vi "单轴运动.vi"() -> ()   [LabVIEW 2011]
uses:
  <userlib>/LTDMC/LTDMC.lvlib
panel:
  in  "停止速度":dbl=100.0
  out "运行曲线图 2":cluster{dbl[], i32[]}[](graph)
  out "运行时间":dbl
  out "当前状态":string
  out "当前速度":dbl
  out "当前位置":i32
  out "运行曲线图":cluster{dbl[], dbl[]}[](graph)
  in  "在线变位":bool
  in  "变位的位置值":i32=21000
  in  "S段时间s":dbl
  in  "减速时间s":dbl=0.5
  in  "加速时间s":dbl=0.5
  in  "运行速度":dbl=100000.0
  in  "起始速度":dbl=500.0
  in  "变速的速度值":dbl=1500.0
  in  "运动模式":enum32{"相对", "绝对"}(radio)
  in  "运动距离":i32=300000
  in  "运动方式":enum32{"点位", "连续"}(radio)
  in  "运动方向":enum32{"正向", "反向"}(radio)
  in  "在线变速":bool
  in  "退出":bool
  in  "紧急停止":bool
  in  "减速停止":bool
  in  "运行":bool
  in  "轴号选择":enum32{"X轴", "Y轴", "Z轴", "C轴"}(radio)
  in  "脉冲清零":bool
  in  "卡号选择":u16(ring) items=["0", "1"]
  out "init":bool
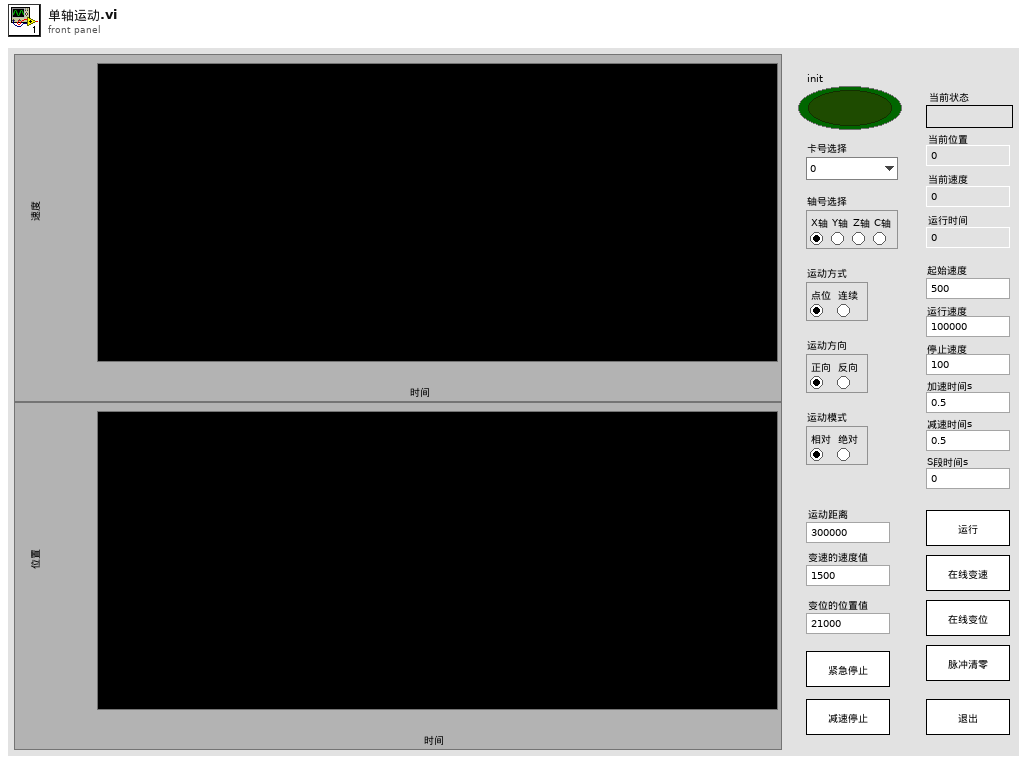
[diagram p1: front panel]
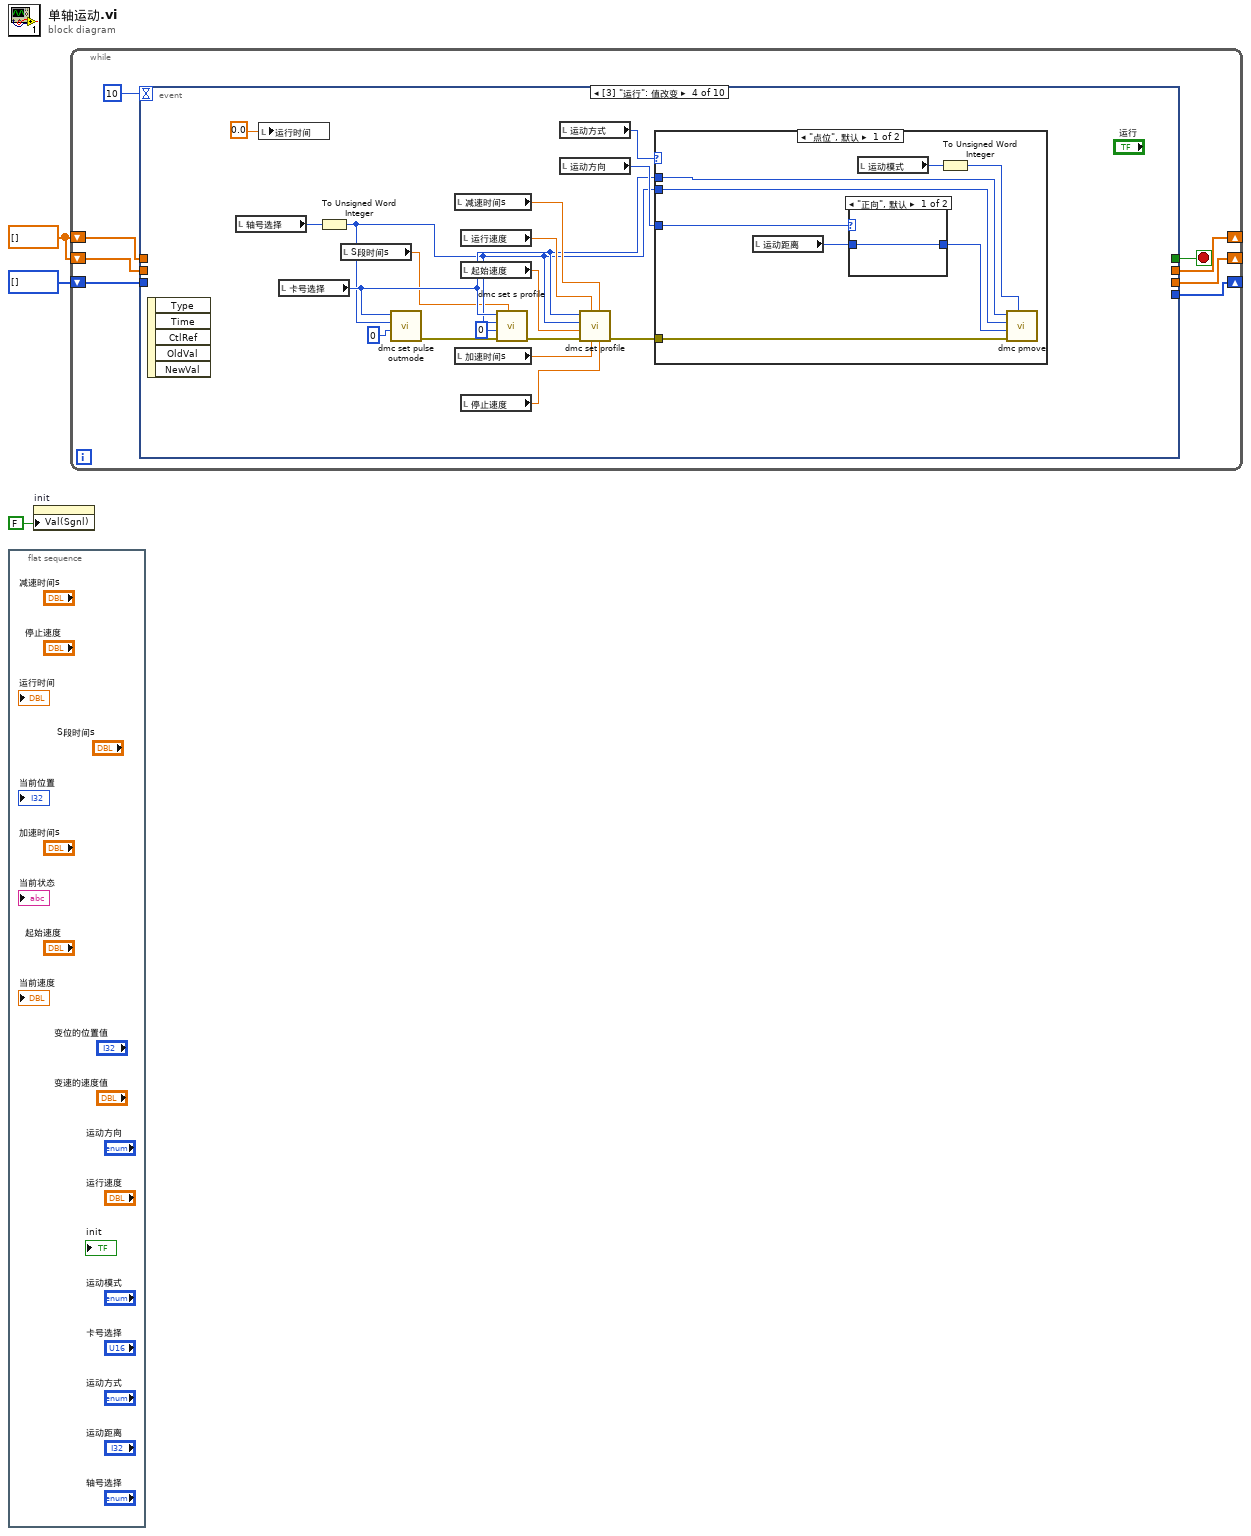
[diagram p0: block diagram]
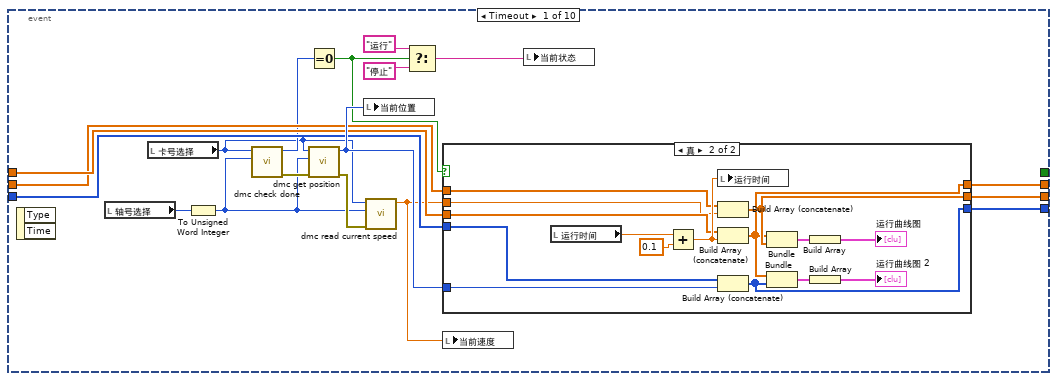
[diagram p2: hidden frame]
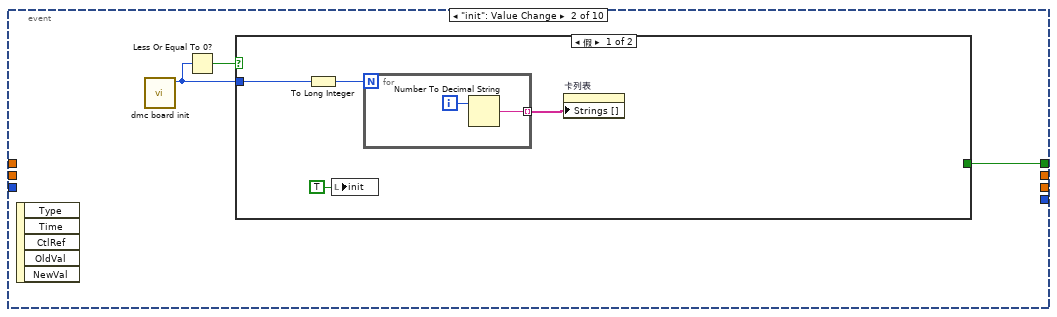
[diagram p4: hidden frame]
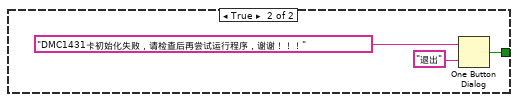
[diagram p5: hidden frame]
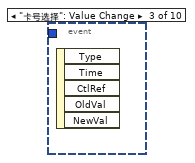
[diagram p6: hidden frame]
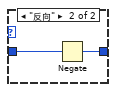
[diagram p7: hidden frame]
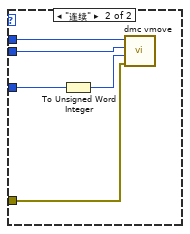
[diagram p8: hidden frame]
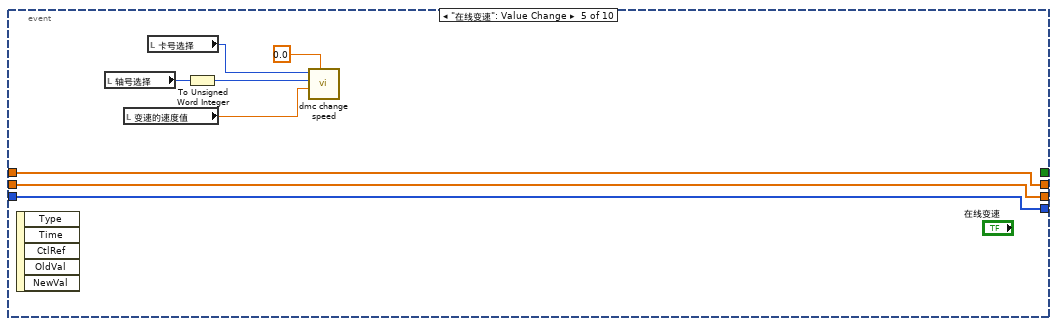
[diagram p9: hidden frame]
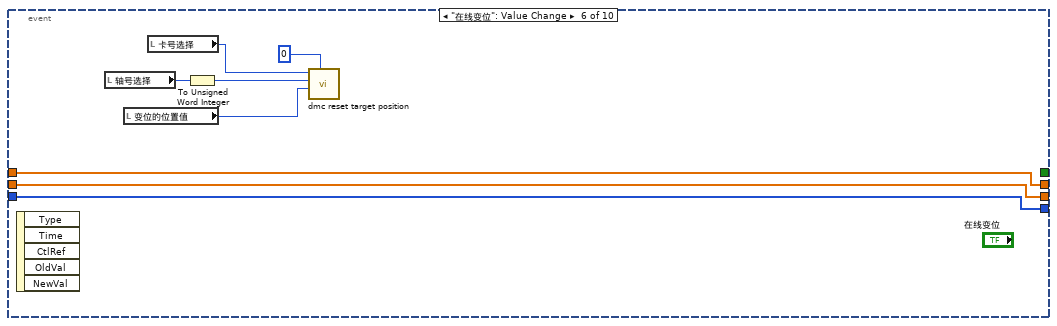
[diagram p10: hidden frame]
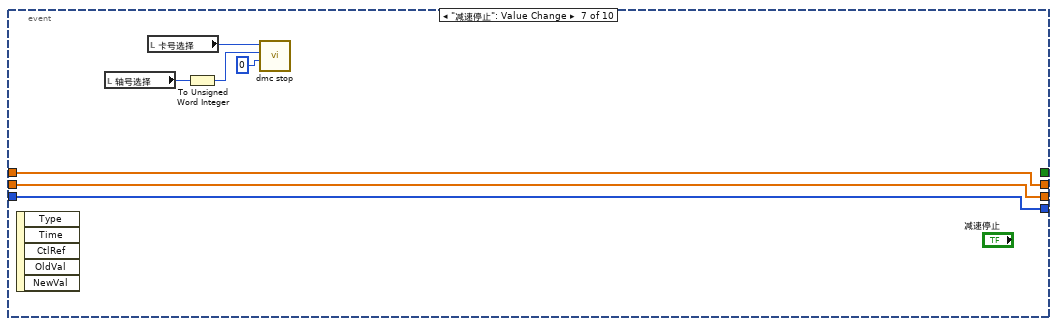
[diagram p11: hidden frame]
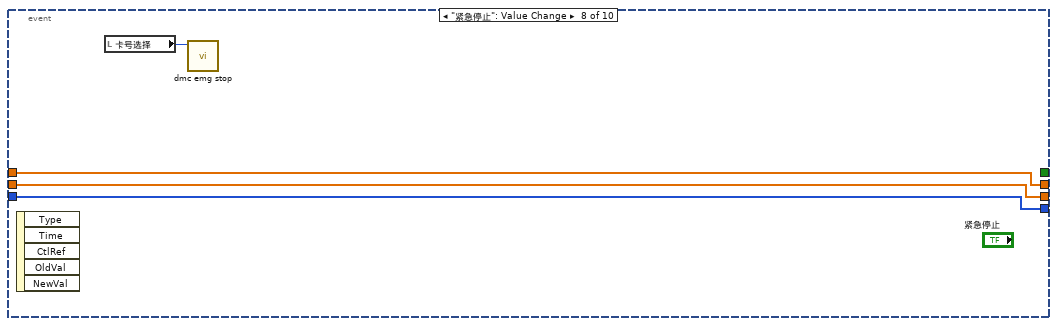
[diagram p12: hidden frame]
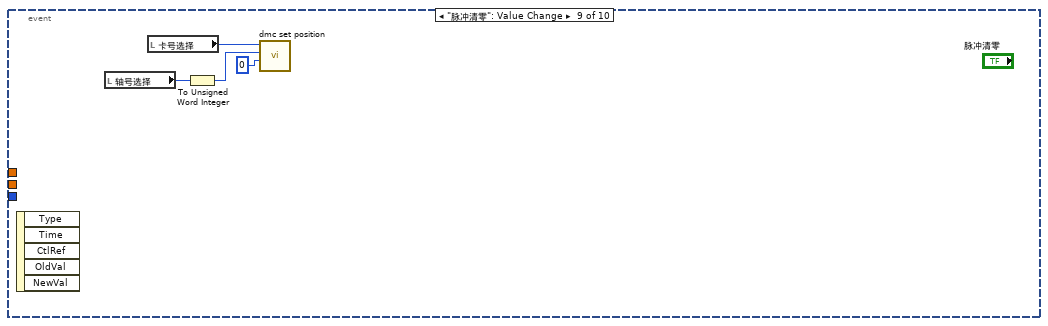
[diagram p13: hidden frame]
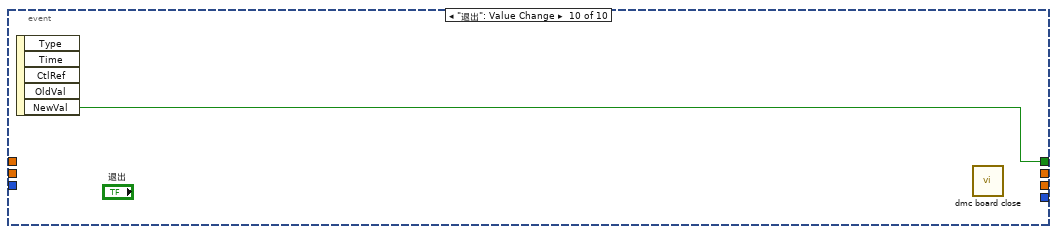
[diagram p14: hidden frame]
diagram:
  w1 = dbl[] []
  n1 = flat-sequence {
    frame #0 {
    }
  }
  n2 = property on="init" class="Bool (严格)"("Val(Sgnl)"=FALSE ("值(信号)")) -> ()  [unwired: 2 in, 2 out]
  n3 = while {
    shift-right: [w9] -> _
    shift-left: w1 -> [w8]
    shift-right: [w7] -> _
    shift-left: i32[] [] -> [w6]
    shift-right: [w4] -> _
    shift-left: w1 -> [w5]
    stop <- w11 stop-if-true
    n4 = event shown="[3] \"运行\": 值改变" {
      selector: _ -> [_ _ _ _ _ _ _ _ _ _]
      dyn-events: _ -> [_ _ _ _ _ _ _ _ _ _]
      timeout: 10 -> [_ _ _ _ _ _ _ _ _ _]
      tunnel: [_ w46 _ _ _ _ _ _ _ w121] -> w11
      tunnel: [w24 _ _ _ w96 w104 w111 w116 _ _] -> w9
      tunnel: w8 -> [w23 _ _ _ w96 w104 w111 w116 _ _]
      tunnel: [w22 _ _ _ w95 w103 w110 w115 _ _] -> w7
      tunnel: w6 -> [w21 _ _ _ w95 w103 w110 w115 _ _]
      tunnel: w5 -> [w20 _ _ _ w94 w102 w109 w114 _ _]
      tunnel: [w19 _ _ _ w94 w102 w109 w114 _ _] -> w4
      event Timeout {
        n5 = event-data() -> ()  [unwired: 1 in, 2 out]
        n6 = local read "轴号选择"() -> (w29:enum32{"X轴", "Y轴", "Z轴", "C轴"})
        n7 = local read "卡号选择"() -> (w13:u16)
        n8 = To Unsigned Word Integer(number=w29) -> (unsigned 16bit integer=w12:u16)
        n9 = call "dmc check done.vi"("axis"=w12, "CardNo"=w13) -> ("error out"=w15:errorcluster, "function return"=w16:i16)  [unwired: 8 in]
        n10 = Equal To 0?(x=w16) -> (x = 0?=w17:bool)
        n11 = call "dmc get position.vi"("error in (no error)"=w15, "axis"=w12, "CardNo"=w13) -> ("error out"=w14:errorcluster, "function return"=w25:i32)  [unwired: 7 in]
        n12 = local write "当前位置"(w25) -> ()
        n13 = call "dmc read current speed.vi"("error in (no error)"=w14, "axis"=w12, "CardNo"=w13) -> ("function return"=w18:dbl)  [unwired: 7 in, 1 out]
        n14 = Select(t="运行" ("当前状态"), s=w17, f="停止" ("当前状态")) -> (s? t:f=w28:string)
        n15 = case shown="真" w17 {
          tunnel: w25 -> [_ w40]
          tunnel: [_ w34] -> w24
          tunnel: w23 -> [_ w41]
          tunnel: [_ w38] -> w22
          tunnel: w21 -> [_ w39]
          tunnel: w20 -> [_ w37]
          tunnel: [_ w35] -> w19
          tunnel: w18 -> [_ w36]
          frame False {
          }
          frame True {
            n16 = local read "运行时间"() -> (w44:dbl)
            n17 = Add(x=w44, y=0.1) -> (x+y=w42:dbl)
            n18 = local write "运行时间"(w42) -> ()
            n19 = Build Array (concatenate)(w37, w36) -> (w35:dbl[])
            n20 = Build Array (concatenate)(w41, w42) -> (w34:dbl[])
            n21 = Build Array (concatenate)(w39, w40) -> (w38:i32[])
            n22 = Bundle(w34, w35) -> (w33:cluster{dbl[], dbl[]})  [unwired: 1 in]
            n23 = Bundle(w34, w38) -> (w30:cluster{dbl[], i32[]})  [unwired: 1 in]
            n24 = Build Array(w33) -> (→"运行曲线图":cluster{dbl[], dbl[]}[])
            n25 = Build Array(w30) -> (→"运行曲线图 2":cluster{dbl[], i32[]}[])
          }
        }
        n26 = local write "当前速度"(w18) -> ()
        n27 = local write "当前状态"(w28) -> ()
      }
      event "init": Value Change {
        n28 = event-data() -> ()  [unwired: 1 in, 5 out]
        n29 = call "dmc board init.vi"() -> ("function return"=w45:i16)  [unwired: 10 in, 1 out]
        n30 = Less Or Equal To 0?(x=w45) -> (x <= 0?=w47:bool)
        n31 = case shown="假" w47 {
          tunnel: [_ w54] -> w46
          tunnel: w45 -> [w51 _]
          frame False {
            n32 = To Long Integer(number=w51) -> (32bit integer=w50:i32)
            n33 = local write "init"(TRUE ("init")) -> ()
            n34 = for {
              N: w50 -> [_]
              tunnel: [w52] -> w49 mode=indexing
              i -> [w53]
              n35 = Number To Decimal String(number=w53) -> (decimal integer string=w52:string)  [unwired: 1 in]
            }
            n36 = property on="卡列表" class="Ring (严格)"("Strings []"=w49) -> ()  [unwired: 2 in, 2 out]
          }
          frame True {
            n37 = One Button Dialog(message="DMC1431卡初始化失败，请检查后再尝试运行程序，谢谢！！！" ("消息"), button name ("OK")="退出" ("按钮名称（“确定”）")) -> (true=w54:bool)
          }
        }
      }
      event "卡号选择": Value Change {
        n38 = event-data() -> ()  [unwired: 1 in, 5 out]
      }
      event "运行": Value Change {
        n39 = event-data() -> ()  [unwired: 1 in, 5 out]
        n40 = local read "轴号选择"() -> (w73:enum32{"X轴", "Y轴", "Z轴", "C轴"})
        n41 = local write "运行时间"(0.0 ("运行时间")) -> ()
        n42 = local read "卡号选择"() -> (w60:u16)
        n43 = To Unsigned Word Integer(number=w73) -> (unsigned 16bit integer=w59:u16)
        n44 = local read "S段时间s"() -> (w58:dbl)
        n45 = call "dmc set pulse outmode.vi"("outmode"=u16 0, "axis"=w59, "CardNo"=w60) -> ("error out"=w66:errorcluster)  [unwired: 7 in, 1 out]
        n46 = local read "减速时间s"() -> (w62:dbl)
        n47 = local read "加速时间s"() -> (w61:dbl)
        n48 = local read "运行速度"() -> (w63:dbl)
        n49 = local read "起始速度"() -> (w64:dbl)
        n50 = local read "停止速度"() -> (w69:dbl)
        n51 = call "dmc set s profile.vi"("s_para"=w58, "error in (no error)"=w66, "s_mode"=u16 0, "axis"=w59, "CardNo"=w60) -> ("error out"=w65:errorcluster)  [unwired: 5 in, 1 out]
        n52 = local read "运动方式"() -> (w72:enum32{"点位", "连续"})
        n53 = local read "运动方向"() -> (w71:enum32{"正向", "反向"})
        n54 = call "dmc set profile.vi"("stop_vel"=w69, "Tdec"=w62, "Tacc"=w61, "Max_Vel"=w63, "error in (no error)"=w65, "Min_Vel"=w64, "axis"=w59, "CardNo"=w60) -> ("error out"=w68:errorcluster)  [unwired: 2 in, 1 out]
        n55 = case shown="\"点位\", 默认" w72 {
          tunnel: w71 -> [w80 w89]
          tunnel: w68 -> [w74 w86]
          tunnel: w59 -> [w78 w85]
          tunnel: w60 -> [w77 w88]
          frame "点位", Default {
            n56 = local read "运动距离"() -> (w79:i32)
            n57 = case shown="\"正向\", 默认" w80 {
              tunnel: w79 -> [w82 w84]
              tunnel: [w82 w83] -> w76
              frame "正向", Default {
              }
              frame "反向" {
                n58 = Negate(x=w84) -> (-x=w83:i32)
              }
            }
            n59 = local read "运动模式"() -> (w81:enum32{"相对", "绝对"})
            n60 = To Unsigned Word Integer(number=w81) -> (unsigned 16bit integer=w75:u16)
            n61 = call "dmc pmove.vi"("posi_mode"=w75, "error in (no error)"=w74, "dist"=w76, "axis"=w78, "CardNo"=w77) -> ()  [unwired: 5 in, 2 out]
          }
          frame "连续" {
            n62 = To Unsigned Word Integer(number=w89) -> (unsigned 16bit integer=w87:u16)
            n63 = call "dmc vmove.vi"("error in (no error)"=w86, "dir"=w87, "axis"=w85, "CardNo"=w88) -> ()  [unwired: 6 in, 2 out]
          }
        }
      }
      event "在线变速": Value Change {
        n64 = event-data() -> ()  [unwired: 1 in, 5 out]
        n65 = local read "轴号选择"() -> (w97:enum32{"X轴", "Y轴", "Z轴", "C轴"})
        n66 = local read "变速的速度值"() -> (w91:dbl)
        n67 = local read "卡号选择"() -> (w92:u16)
        n68 = To Unsigned Word Integer(number=w97) -> (unsigned 16bit integer=w93:u16)
        n69 = call "dmc change speed.vi"("Taccdec"=0.0, "Curr_Vel"=w91, "axis"=w93, "CardNo"=w92) -> ()  [unwired: 6 in, 2 out]
      }
      event "在线变位": Value Change {
        n70 = event-data() -> ()  [unwired: 1 in, 5 out]
        n71 = local read "轴号选择"() -> (w105:enum32{"X轴", "Y轴", "Z轴", "C轴"})
        n72 = local read "变位的位置值"() -> (w99:i32)
        n73 = local read "卡号选择"() -> (w101:u16)
        n74 = To Unsigned Word Integer(number=w105) -> (unsigned 16bit integer=w100:u16)
        n75 = call "dmc reset target position.vi"("posi_mode"=u16 0, "dist"=w99, "axis"=w100, "CardNo"=w101) -> ()  [unwired: 6 in, 2 out]
      }
      event "减速停止": Value Change {
        n76 = event-data() -> ()  [unwired: 1 in, 5 out]
        n77 = local read "轴号选择"() -> (w112:enum32{"X轴", "Y轴", "Z轴", "C轴"})
        n78 = local read "卡号选择"() -> (w106:u16)
        n79 = To Unsigned Word Integer(number=w112) -> (unsigned 16bit integer=w107:u16)
        n80 = call "dmc stop.vi"("stop_mode"=u16 0, "axis"=w107, "CardNo"=w106) -> ()  [unwired: 7 in, 2 out]
      }
      event "紧急停止": Value Change {
        n81 = event-data() -> ()  [unwired: 1 in, 5 out]
        n82 = local read "卡号选择"() -> (w113:u16)
        n83 = call "dmc emg stop.vi"("CardNo"=w113) -> ()  [unwired: 9 in, 2 out]
      }
      event "脉冲清零": Value Change {
        n84 = event-data() -> ()  [unwired: 1 in, 5 out]
        n85 = local read "轴号选择"() -> (w120:enum32{"X轴", "Y轴", "Z轴", "C轴"})
        n86 = local read "卡号选择"() -> (w119:u16)
        n87 = To Unsigned Word Integer(number=w120) -> (unsigned 16bit integer=w118:u16)
        n88 = call "dmc set position.vi"("current_position"=0, "axis"=w118, "CardNo"=w119) -> ()  [unwired: 7 in, 2 out]
      }
      event "退出": Value Change {
        n89 = event-data() -> ("NewVal"=w121:bool)  [unwired: 1 in, 4 out]
        n90 = call "dmc board close.vi"() -> ()  [unwired: 10 in, 2 out]
      }
    }
  }
